vi "TPND_DefaultMail.vi"(5 "host name":string, 6 "device":string, 7 "user":string, 9 "application name":string, 10 "alarm message":string, 11 "next alarm":dbl) -> (2 "mail out":string)   [LabVIEW 2016]
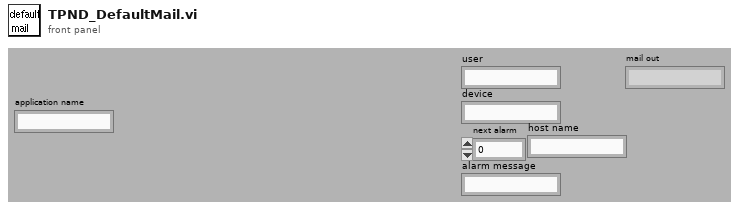
[diagram p1: front panel]
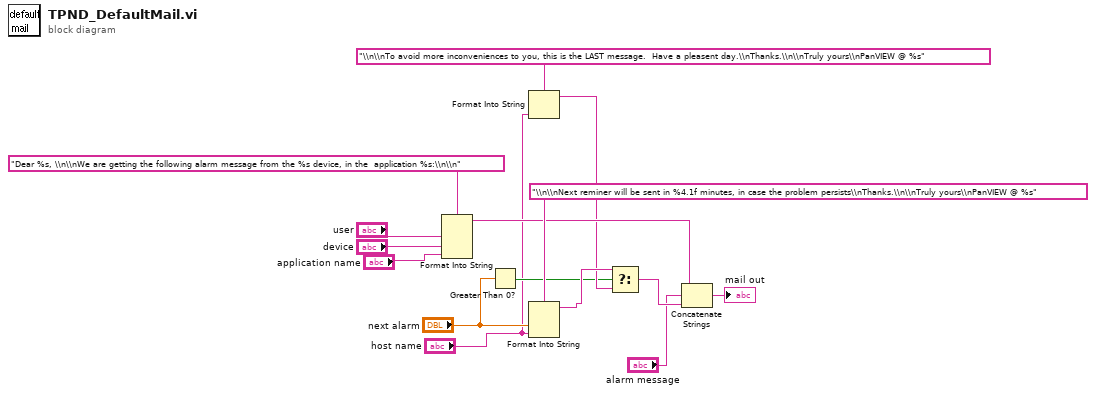
[diagram p0: block diagram]
diagram:
  n1 = Format Into String(format string="Dear %s, \\n\\nWe are getting the following alarm message from the %s device, in the  application %s:\\n\\n", "user", "device", "application name") -> (resulting string=w13:string)  [unwired: 2 in, 1 out]
  n2 = Greater Than 0?(x="next alarm") -> (x > 0?=w4:bool)
  n3 = Format Into String(format string="\\n\\nTo avoid more inconveniences to you, this is the LAST message.  Have a pleasent day.\\nThanks.\\n\\nTruly yours\\nPanVIEW @ %s", "host name") -> (resulting string=w10:string)  [unwired: 2 in, 1 out]
  n4 = Format Into String(format string="\\n\\nNext reminer will be sent in %4.1f minutes, in case the problem persists\\nThanks.\\n\\nTruly yours\\nPanVIEW @ %s", "next alarm", "host name") -> (resulting string=w12:string)  [unwired: 2 in, 1 out]
  n5 = Select(t=w12, s=w4, f=w10) -> (s? t:f=w11:string)
  n6 = Concatenate Strings(w13, "alarm message", w11) -> (→"mail out":string)
